vi "Set AO Graph Y Axis (WFGraph).vi"(8 "error in (no error)":errorcluster, 10 "Y Axis (Output)":enum16{"Analog Output", "Reference"}(ring) caption="Enum 3", 11 "WaveformGraph in":refnum<vi>) -> (0 "error out":errorcluster)   [LabVIEW 2019, in "Instrument.Lockin.UI.lvclass"]
uses:
  Instrument.Lockin.UI.lvclass
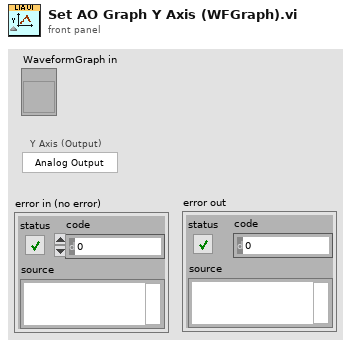
[diagram p1: front panel]
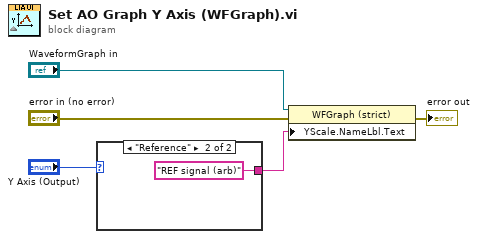
[diagram p0: block diagram]
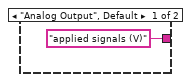
[diagram p2: hidden frame]
diagram:
  n1 = case shown="\"Reference\"" "Y Axis (Output)" {
    tunnel: ["applied signals (V)" ("Y Scale.Name Label.Text") "REF signal (arb)" ("Y Scale.Name Label.Text")] -> w1
    frame "Analog Output", Default {
    }
    frame "Reference" {
    }
  }
  n2 = property on="Property Node" class="WFGraph (strict)"(reference="WaveformGraph in", error in="error in (no error)", "YScale.NameLbl.Text"=w1) -> (error out=→"error out":errorcluster)  [unwired: 1 out]
